vi "Simulator_0720.vi"() -> ()   [LabVIEW 2017]
doc: "This example demonstrates how to continuously acquire buffered voltage measurements using a DAQmx device.\n\nFor instructions on how to connect your signals to the DAQ device, refer to your device documentation."
uses:
  <vilib>/Utility/error.llb/DialogType.ctl
  <vilib>/DAQmx/read.llb/DAQmx Read (Analog 1D Wfm NChan NSamp).vi
  <vilib>/Analysis/5stat.llb/RMS (DBL).vi
  <vilib>/DAQmx/miscellaneous.llb/DAQmx Fill In Error Info.vi
  <vilib>/express/express shared/transition.llb/Dynamic To Waveform Array.vi
  <vilib>/express/express arith-compare/Formula/Block/exnFormulaBlock how many pts in the wave.vi
  <vilib>/express/express shared/ex_Modify Signal Name.vi
  <vilib>/express/express shared/transition.llb/Waveform Array To Dynamic.vi
  <vilib>/measure/maspectr.llb/FFT Power Spectrum and PSD for N Chan.vi
  <vilib>/measure/mascope.llb/Cycle Average and RMS N chan.vi
  <vilib>/express/express arith-compare/Formula/XNode/ExpressFormulaBlockNode.xnode
  <vilib>/measure/NI_MAPro.lvlib
  SetupDAQ.vi
  <vilib>/Analysis/NI_AALPro.lvlib
  <vilib>/ptbypt/NI_PtbyPt.lvlib
panel:
  out "A,B,C,D Filtering Signal 5":dbl(graph) caption="A,B Filtering Signal"
  out "Raw Signal 4":dynamicdata(graph)
  out "Raw Signal 3":waveform(dbl)[](graph)
  out "A,B,C,D Filtering Signal 4":dbl(graph) caption="A,B Filtering Signal"
  out "A,B,C,D Filtering Signal 3":dynamicdata(graph) caption="A,B Filtering Signal"
  out "A,B,C,D Filtering Signal 2":dynamicdata(graph) caption="A,B Filtering Signal"
  out "슬라이드 2":dbl(slide) scale=-0.6..3.0
  out "슬라이드":dbl(slide) scale=1.0..3.5
  out "2.5HZ-Step":dynamicdata(graph)
  in  "동작 라벨":T1(radio)
  in  "Sensor C Channel 2":tag="Dev2/ai0"
  in  "Sensor D Channel 2":tag="Dev2/ai1"
  in  "Terminal config 2":i32(ring)=10083 items=["default"=-1, "RSE"=10083, "NRSE"=10078, "Differential"=10106, "Pseudodifferential"=12529]
  out "55-65(A)":dynamicdata(graph)
  out "10-20(A)":dynamicdata(graph)
  out "A,B,C,D Filtering Signal":dynamicdata(graph) caption="A,B Filtering Signal"
  out "Differential Signal A-B, C-D":dynamicdata(graph)
  in  "number of averages":u32=1
  out "Power Spectrum / PSD":cluster{"f0":dbl, "df":dbl, "magnitude":dbl[]}[](graph)
  out "detected amplitudes 2":dbl(graph)=1.1331379876254155
  out "detected frequencies 2":dbl(graph)
  out "detected frequencies":dbl[](array[numeric])=[60.0, 60.0]
  out "detected amplitudes":dbl[](array[numeric])=[1.1331379876254155, 0.40633237156802526]
  out "Raw Signal 2":waveform(dbl)[](graph)
  out "Raw Signal":waveform(dbl)[](graph)
  in  "Sensor B Channel":tag="Dev2/ai1"
  in  "Sensor A Channel":tag="Dev2/ai0"
  in  "Terminal config":i32(ring)=10083 items=["default"=-1, "RSE"=10083, "NRSE"=10078, "Differential"=10106, "Pseudodifferential"=12529]
  in  "rate":dbl=5000.0
  out "FFT Power Spectrum":cluster{"f0":dbl, "df":dbl, "magnitude":dbl[]}[](graph)
  in  "Stop":bool
  in  "Number of Samples":i32=100
  # "Channel Settings"
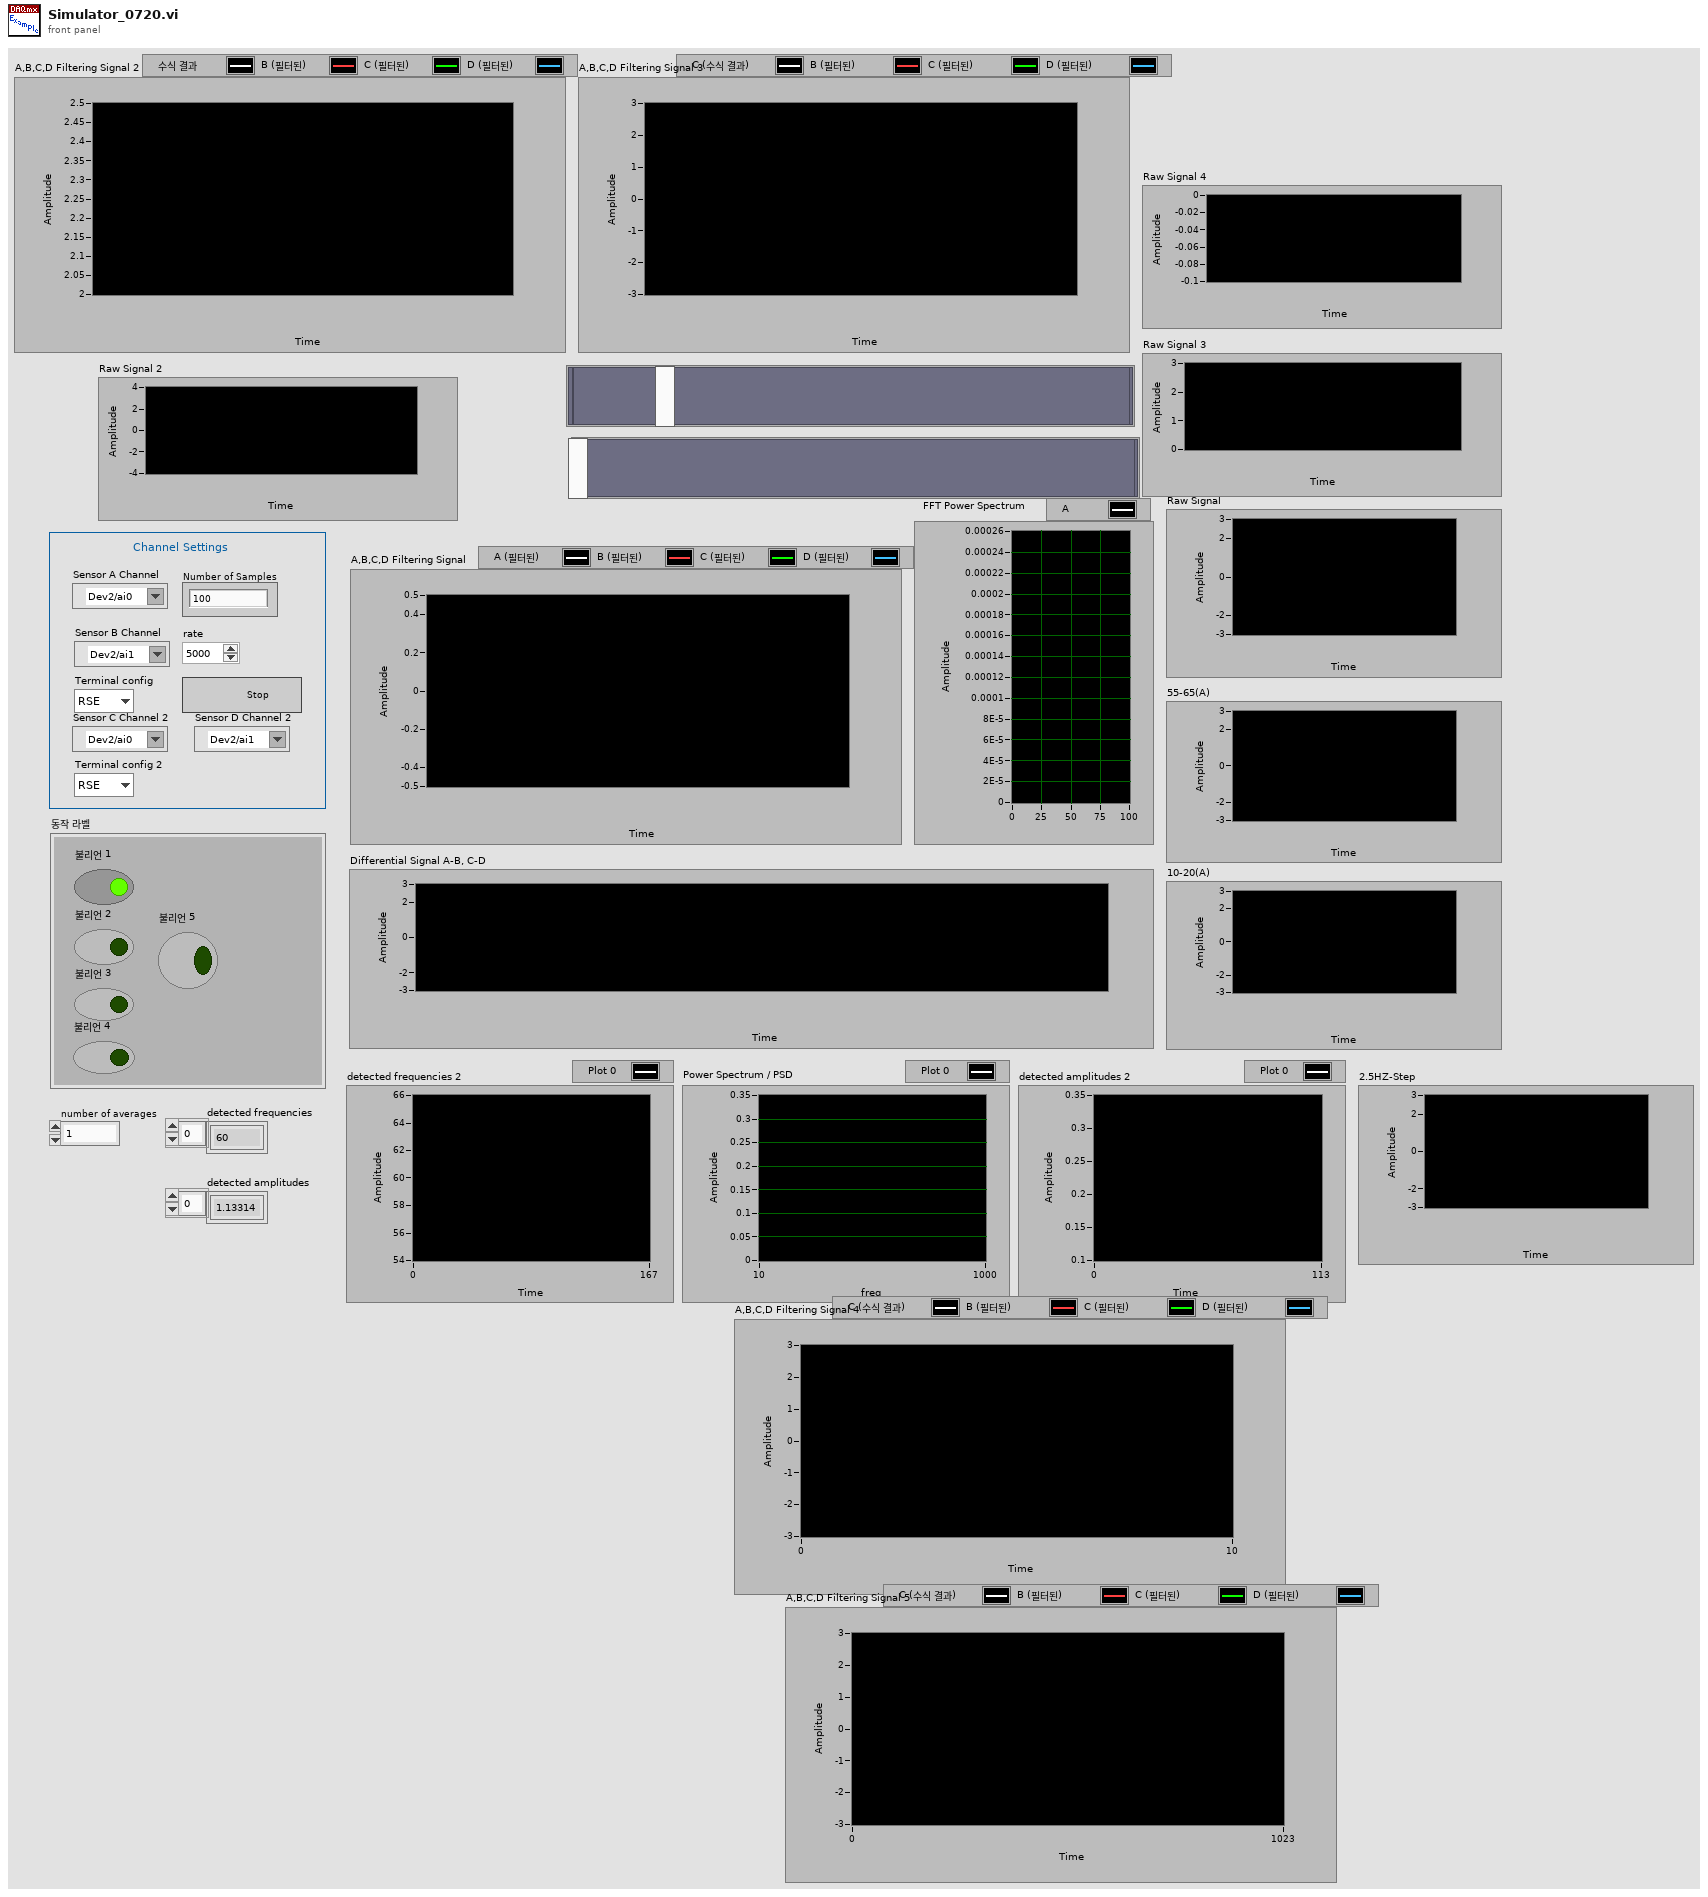
[diagram p1: front panel]
types:
  T1 = enum32{"불리언 1", "불리언 2", "불리언 3", "불리언 4", "불리언 5"}
  T2 = typedef "DialogType.ctl" = u16
  T3 = cluster{"averaging mode":enum16{"No averaging", "Vector averaging", "RMS averaging", "Peak hold"}, "weighting mode":enum16{"Linear", "Exponential"}, "number of averages":u32}
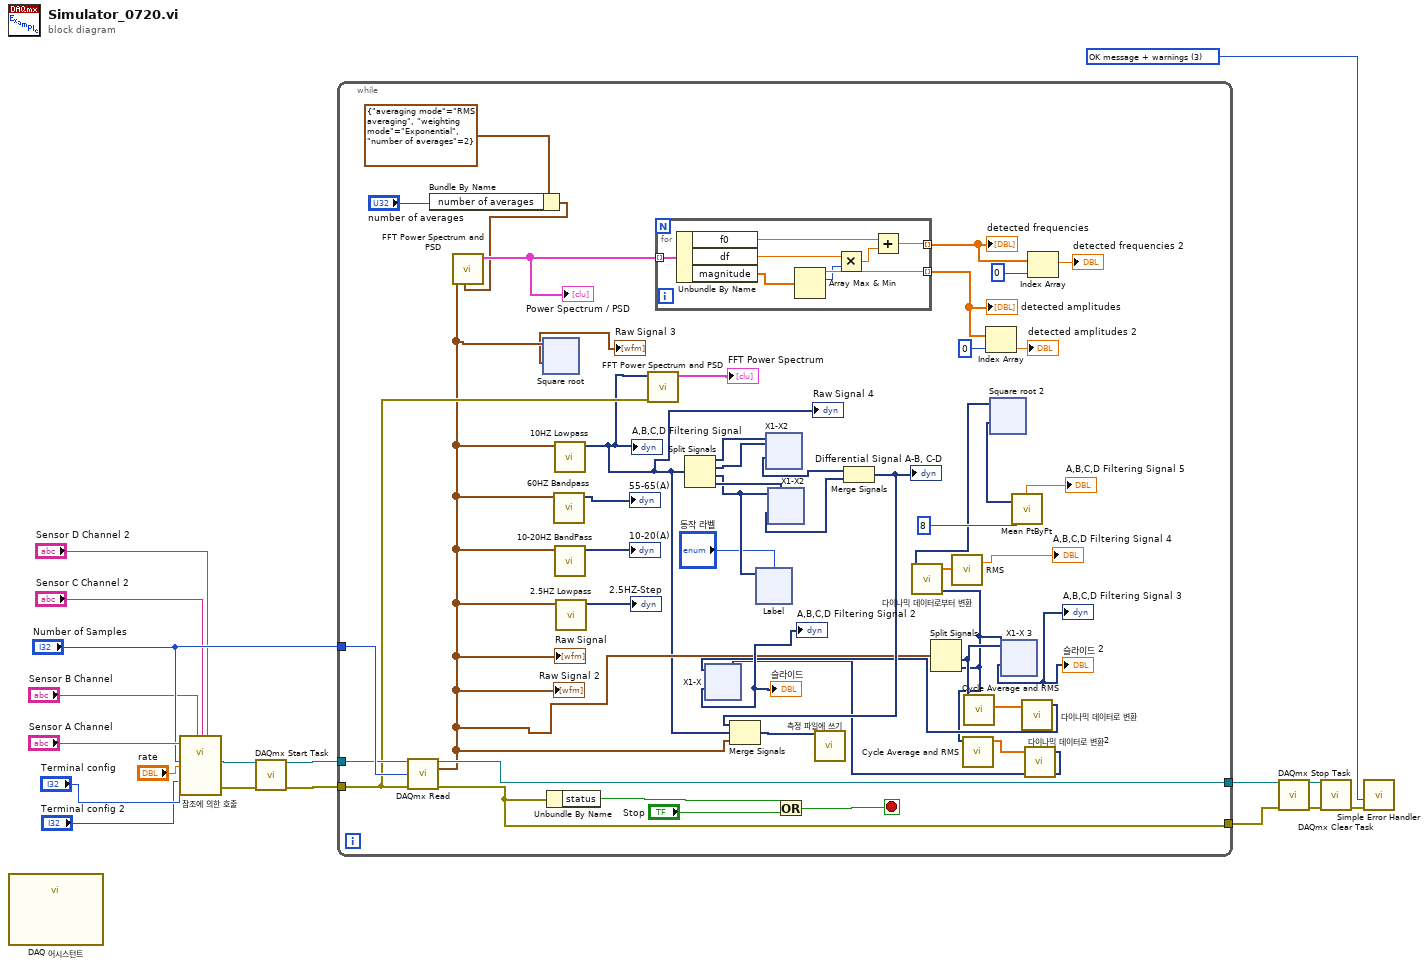
[diagram p0: block diagram]
diagram:
  w11 = T2 3 items=["no dialog", "OK message", "continue or stop message", "OK message + warnings", "continue/stop + warnings"] ("type of dialog (OK msg:1)")
  n1 = call "DAQ 어시스턴트"() -> ()  [unwired: 12 in]
  n2 = call-by-ref "참조에 의한 호출"("number of samples"="Number of Samples", "rate"="rate", "input terminal configuration"="Terminal config", "input terminal configuration 2"="Terminal config 2", "physical channel"="Sensor A Channel", "physical channel 2"="Sensor B Channel", "physical channel 3"="Sensor C Channel 2", "physical channel 4"="Sensor D Channel 2") -> ("task out"=w7:refnum<k21>, "error out"=w6:errorcluster)  [unwired: 12 in, 2 out]
  n3 = call <vilib>:"DAQmx Start Task.vi"("task/channels in"=w7, "error in"=w6) -> ("task out"=w18:refnum<k21>, "error out"=w17:errorcluster)  [unwired: 12 in]
  n4 = while "While 루프" {
    tunnel: w18 -> [w60]
    tunnel: w17 -> [w59]
    tunnel: [w65] -> w15
    tunnel: [w63] -> w14
    tunnel: "Number of Samples" -> [w61]
    stop <- w62 stop-if-true
    n5 = call-poly <vilib>:"DAQmx Read.vi"("task/channels in"=w60, "number of samples per channel"=w61, "error in"=w59) -> ("task out"=w65:refnum<k21>, "data"=w25:waveform(dbl)[], "error out"=w63:errorcluster)  [unwired: 10 in]
    "Raw Signal" <- w25
    "Raw Signal 2" <- w25
    n6 = Bundle By Name ("이름으로 묶기")(cluster=T3 {"averaging mode"=enum."RMS averaging", "weighting mode"=enum."Exponential", "number of averages"=2} ("averaging parameters"), "number of averages"="number of averages") -> (w35:T3)
    n7 = call-poly <vilib>:"FFT Power Spectrum and PSD.vi"("averaging parameters"=w35, "time signals"=w25) -> ("Power Spectrum / PSD"=w37:cluster{"f0":dbl, "df":dbl, "magnitude":dbl[]}[])  [unwired: 6 in, 3 out]
    "Power Spectrum / PSD" <- w37
    n8 = xnode "Square root"("X1"=w25) -> ("결과"=→"Raw Signal 3":waveform(dbl)[])  [unwired: 1 in, 1 out]
    n9 = Unbundle By Name(w63) -> ("status"=w50:bool)
    n10 = call "60HZ Bandpass"("Signal"=w25) -> ("Filtered Signal"=→"55-65(A)":dynamicdata)  [unwired: 9 in, 1 out]
    n11 = call "10HZ Lowpass"("Signal"=w25) -> ("Filtered Signal"=w23:dynamicdata)  [unwired: 9 in, 1 out]
    "A,B,C,D Filtering Signal" <- w23
    "Raw Signal 4" <- w23
    n12 = call "10-20HZ BandPass"("Signal"=w25) -> ("Filtered Signal"=→"10-20(A)":dynamicdata)  [unwired: 9 in, 1 out]
    n13 = call "2.5HZ Lowpass"("Signal"=w25) -> ("Filtered Signal"=→"2.5HZ-Step":dynamicdata)  [unwired: 9 in, 1 out]
    n14 = call-poly <vilib>:"FFT Power Spectrum and PSD.vi"("error in (no error)"=w59, "time signals"=w23) -> ("Power Spectrum / PSD"=→"FFT Power Spectrum":cluster{"f0":dbl, "df":dbl, "magnitude":dbl[]}[])  [unwired: 6 in, 3 out]
    n15 = for {
      tunnel: w37 -> [w904] mode=indexing
      tunnel: [w907] -> w56 mode=indexing
      tunnel: [w905] -> w53 mode=indexing
      n16 = Unbundle By Name(w904) -> ("f0"=w900:dbl, "df"=w906:dbl, "magnitude"=w903:dbl[])
      n17 = Array Max & Min(array=w903) -> (max value=w907:dbl, max index (indices)=w902:i32)  [unwired: 2 out]
      n18 = Multiply(x=w906, y=w902) -> (x*y=w901:dbl)
      n19 = Add(x=w900, y=w901) -> (x+y=w905:dbl)
    }
    "detected amplitudes" <- w56
    "detected frequencies" <- w53
    n20 = Split Signals(w23) -> (w46:dynamicdata, w45:dynamicdata, w41:dynamicdata, w44:dynamicdata)  [unwired: 4 in]
    n21 = xnode "Label"("X1"=w41, "X2"="동작 라벨") -> ()  [unwired: 1 in, 2 out]
    n22 = xnode "X1-X2"("X1"=w46, "X2"=w45) -> ("결과"=w43:dynamicdata)  [unwired: 1 in, 1 out]
    n23 = xnode "X1-X2"("X1"=w41, "X2"=w44) -> ("결과"=w42:dynamicdata)  [unwired: 1 in, 1 out]
    n24 = Or(x=w50, y="Stop") -> (x .or. y?=w62:bool)
    n25 = Merge Signals(w43, w42) -> (w39:dynamicdata)
    "Differential Signal A-B, C-D" <- w39
    n26 = Merge Signals(w39, w23, w25) -> (w38:dynamicdata)
    n27 = call "측정 파일에 쓰기"("Signals"=w38) -> ()  [unwired: 16 in, 3 out]
    n28 = Split Signals(w25) -> (w32:dynamicdata, w20:dynamicdata)  [unwired: 4 in, 2 out]
    n29 = call "다이나믹 데이터로부터 변환"("Dynamic Data Type"=w20) -> ("Array"=w27:dbl[])  [unwired: 3 in]
    n30 = call-poly <vilib>:"RMS.vi"("X"=w27) -> ("rms value"=→"A,B,C,D Filtering Signal 4":dbl)  [unwired: 1 out]
    n31 = call-poly <vilib>:"Cycle Average and RMS.vi"("signal(s) in"=w20) -> ("cycle average"=w29:dbl[])  [unwired: 7 in, 3 out]
    n32 = call-poly <vilib>:"Cycle Average and RMS.vi"("signal(s) in"=w32) -> ("cycle RMS"=w28:dbl[])  [unwired: 7 in, 3 out]
    n33 = Index Array(array=w56, index=0) -> (element=→"detected amplitudes 2":dbl)
    n34 = xnode "Square root 2"("X1"=w20) -> ("결과"=w19:dynamicdata)  [unwired: 1 in, 1 out]
    n35 = xnode "X1-X 3"("X1"=w32, "X2"=w20) -> ("결과"=→"슬라이드 2" →"A,B,C,D Filtering Signal 3":dynamicdata)  [unwired: 1 in, 1 out]
    n36 = call <vilib>:"Mean PtByPt.vi"("x"=w19, "sample length"=8) -> ("mean"=→"A,B,C,D Filtering Signal 5":dbl)  [unwired: 2 in, 1 out]
    n37 = call "다이나믹 데이터로 변환"("Array"=w28) -> ("Dynamic Data Type"=w31:dynamicdata)  [unwired: 3 in]
    n38 = call "다이나믹 데이터로 변환2"("Array"=w29) -> ("Dynamic Data Type"=w30:dynamicdata)  [unwired: 3 in]
    n39 = xnode "X1-X"("X1"=w31, "X2"=w30) -> ("결과"=→"슬라이드" →"A,B,C,D Filtering Signal 2":dynamicdata)  [unwired: 1 in, 1 out]
    n40 = Index Array(array=w53, index=0) -> (element=→"detected frequencies 2":dbl)
  }
  n41 = call <vilib>:"DAQmx Stop Task.vi"("task/channels in"=w15, "error in"=w14) -> ("task out"=w12:refnum<k21>, "error out"=w13:errorcluster)  [unwired: 12 in]
  n42 = call <vilib>:"DAQmx Clear Task.vi"("task in"=w12, "error in"=w13) -> ("error out"=w16:errorcluster)  [unwired: 13 in]
  n43 = call <vilib>:"Simple Error Handler.vi"("type of dialog (OK msg:1)"=w11, "error in (no error)"=w16) -> ()  [unwired: 3 in, 5 out]
